vi "State_Machine.vi"() -> ()   [LabVIEW 2022 SP3]
uses:
  SM_States.ctl
  Database_element.ctl
  SM_Data.ctl
panel:
  out "Database":string
  in  "Add Item":bool
  in  "Exit":bool
  in  "Search":bool
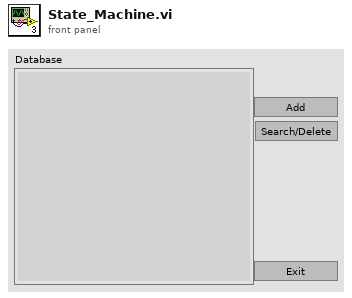
[diagram p1: front panel]
types:
  T1 = typedef "SM_States.ctl" = enum16{"Idle", "Initialize", "Exit", "Update Indicator", "Error Handle", "Delete Item", "Add Item", "Search And Delete"}
  T2 = typedef "Database_element.ctl" = cluster{"Product Number":i32, "Product Name":string, "Manufacturer":string}
  T3 = typedef "SM_Data.ctl" = cluster{"Database":T2[], "Indicator":string}
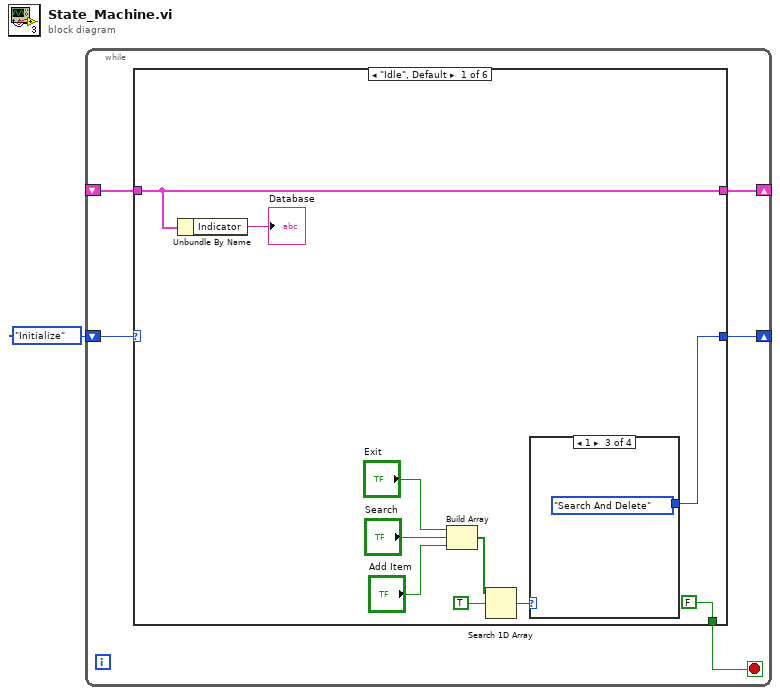
[diagram p0: block diagram]
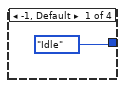
[diagram p2: hidden frame]
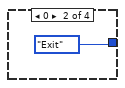
[diagram p3: hidden frame]
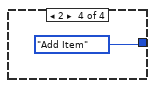
[diagram p4: hidden frame]
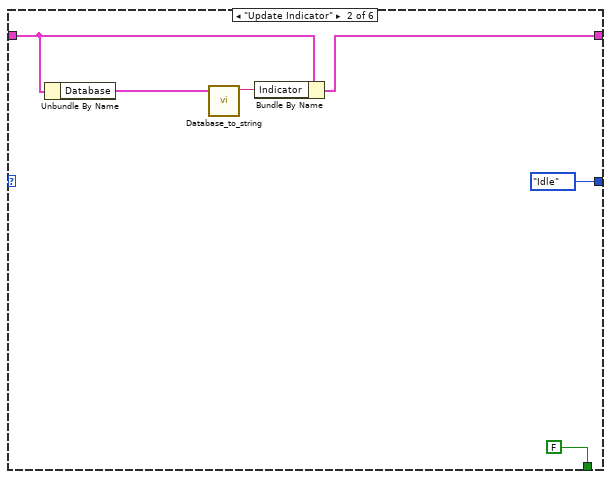
[diagram p5: hidden frame]
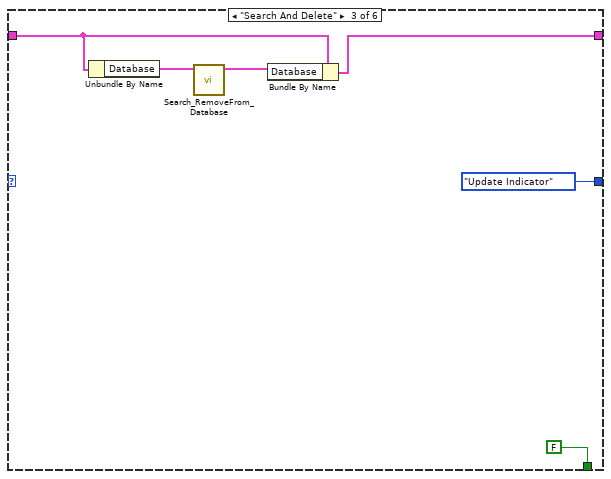
[diagram p6: hidden frame]
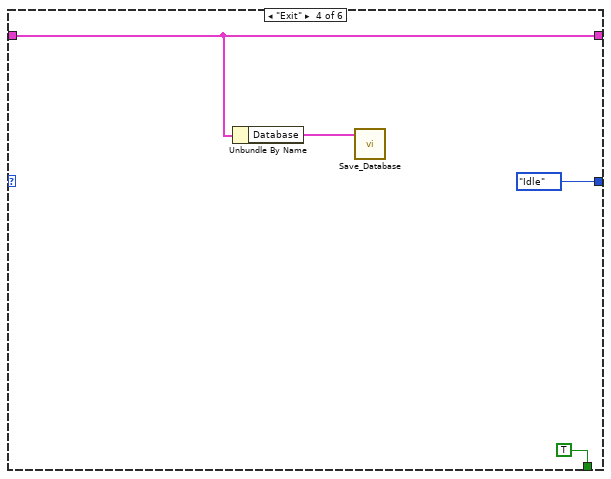
[diagram p7: hidden frame]
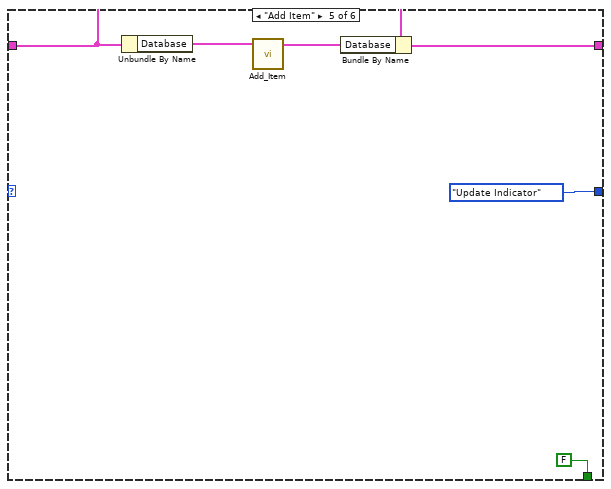
[diagram p8: hidden frame]
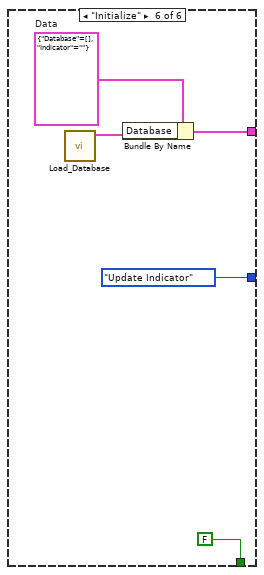
[diagram p9: hidden frame]
diagram:
  n1 = while {
    shift-right: [w5] -> _
    shift-left: SM_States."Initialize" ("States") -> [w6]
    shift-right: [w4] -> _
    shift-left: _ -> [w3]
    stop <- w2 stop-if-true
    n2 = case shown="\"Idle\", Default" w6 {
      tunnel: [w13 SM_States."Idle" ("States") SM_States."Update Indicator" ("States") SM_States."Idle" ("States") SM_States."Update Indicator" ("States") SM_States."Update Indicator" ("States")] -> w5
      tunnel: [w8 w24 w27 w34 w37 w43] -> w4
      tunnel: w3 -> [w8 w25 w28 w34 w39 _]
      tunnel: [FALSE FALSE FALSE TRUE FALSE FALSE] -> w2
      frame "Idle", Default {
        n3 = Unbundle By Name(w8) -> ("Indicator"=→"Database":string)
        n4 = Build Array("Exit", "Search", "Add Item") -> (w11:bool[])
        n5 = Search 1D Array(1D array=w11, element=TRUE) -> (index of element=w12:i32)  [unwired: 1 in]
        n6 = case shown="1" w12 {
          tunnel: [SM_States."Idle" ("States") SM_States."Exit" ("States") SM_States."Search And Delete" ("States") SM_States."Add Item" ("States")] -> w13
          frame -1, Default {
          }
          frame 0 {
          }
          frame 1 {
          }
          frame 2 {
          }
        }
      }
      frame "Update Indicator" {
        n7 = Unbundle By Name(w25) -> ("Database"=w22:T2[])
        n8 = call "Database_to_string.vi"("Array"=w22) -> ("String"=w21:string)  [unwired: 9 in, 1 out]
        n9 = Bundle By Name(cluster=w25, "Indicator"=w21) -> (w24:T3)
      }
      frame "Search And Delete" {
        n10 = Unbundle By Name(w28) -> ("Database"=w30:T2[])
        n11 = call "Search_RemoveFrom_Database.vi"("Database In"=w30) -> ("Database Out"=w29:T2[])  [unwired: 10 in]
        n12 = Bundle By Name(cluster=w28, "Database"=w29) -> (w27:T3)
      }
      frame "Exit" {
        n13 = Unbundle By Name(w34) -> ("Database"=w33:T2[])
        n14 = call "Save_Database.vi"("Database"=w33) -> ()  [unwired: 10 in, 1 out]
      }
      frame "Add Item" {
        n15 = Unbundle By Name(w39) -> ("Database"=w40:T2[])
        n16 = call "Add_Item.vi"("Database"=w40) -> ("Modified Database"=w38:T2[])  [unwired: 9 in, 1 out]
        n17 = Bundle By Name(cluster=w39, "Database"=w38) -> (w37:T3)
      }
      frame "Initialize" {
        w44 = T3 {"Database"=[], "Indicator"=""}  # Data
        n18 = call "Load_Database.vi"() -> ("Database"=w45:T2[])  [unwired: 10 in, 1 out]
        n19 = Bundle By Name(cluster=w44, "Database"=w45) -> (w43:T3)
      }
    }
  }
